vi "CheckGameBoardSnakeCheck.vi"(8 "error in (no error)":errorcluster, 11 "Board in":T3[][](array[typedef])) -> (0 "error out":errorcluster, 1 "positions":T1, 2 "Results":T2, 3 "Board out":T3[][](array[typedef]))   [LabVIEW 2020]
uses:
  TypeDef/tiles-key-trunct.ctl
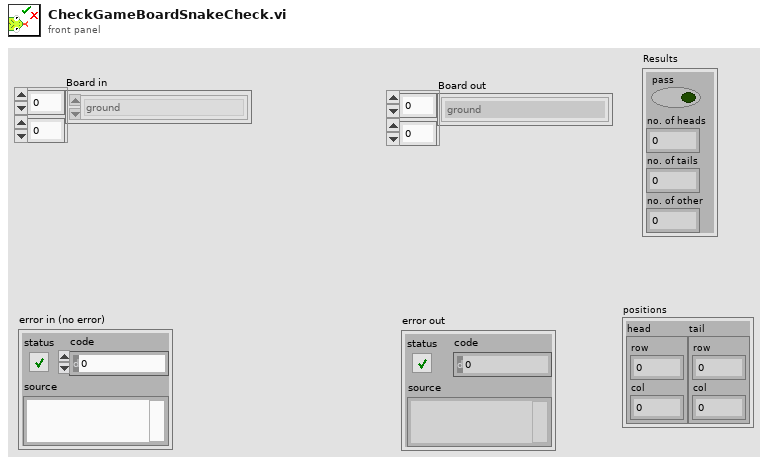
[diagram p1: front panel]
types:
  T1 = cluster{"head":cluster{"row":i32, "col":i32}, "tail":cluster{"row":i32, "col":i32}}
  T2 = cluster{"pass":bool, "no. of heads":i32, "no. of tails":i32, "no. of other":i32}
  T3 = typedef "tiles-key-trunct.ctl" = enum16{"ground", "wall", "head (right)", "head (up)", "head (left)", "head (down)", "L-turn (right-up)", "L-turn (up-left)", "L-turn (left-down)", "L-turn (down-right)", "body (right)", "body (up)", "body (left)", "body (down)", "R-turn (right-down)", "R-turn (up-right)", "R-turn (left-up)", "R-turn (down-left)", "tail (right)", "tail (up)", "tail (left)", "tail (down)"}
  T4 = typedef "direction.ctl" = enum16{"Right", "Up", "Left", "Down"}
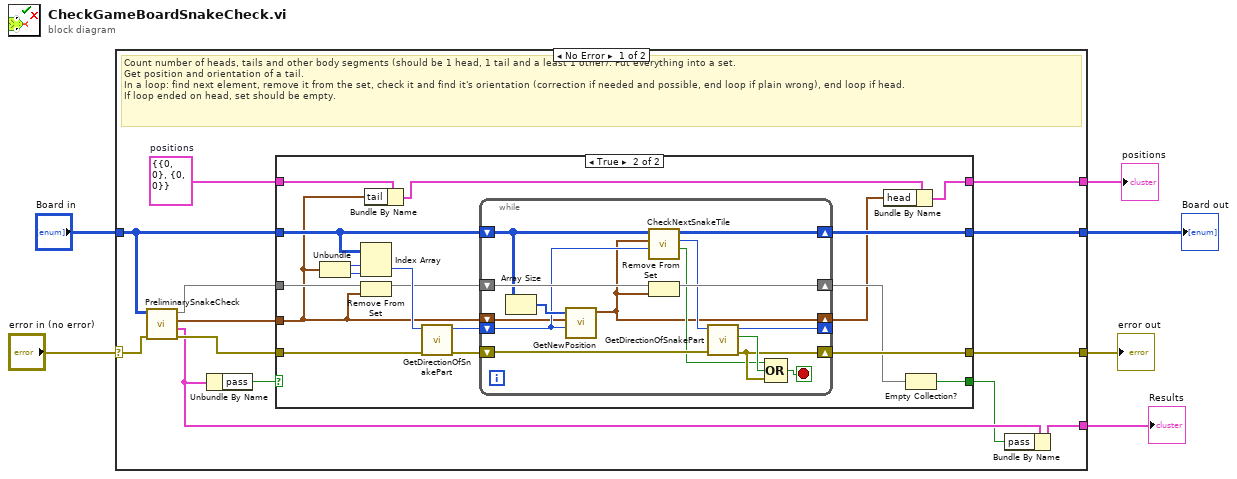
[diagram p0: block diagram]
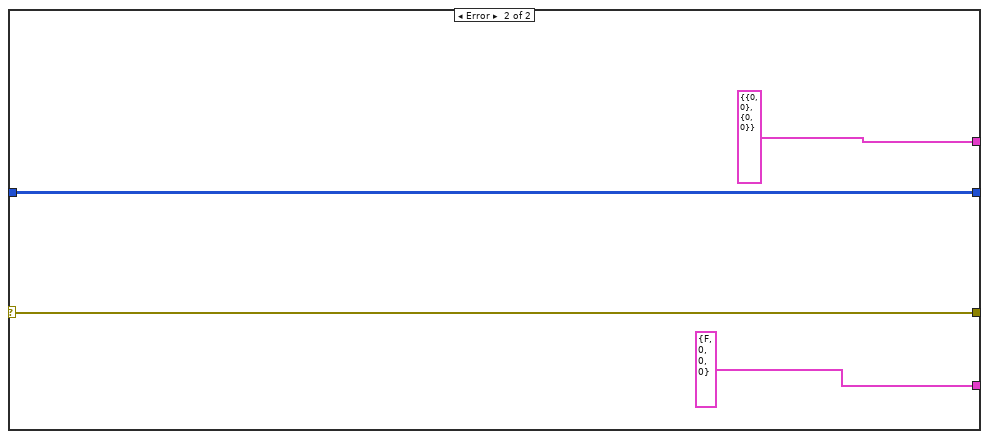
[diagram p3: hidden frame]
diagram:
  n1 = case shown="No Error" "error in (no error)" {
    selector: "error in (no error)" -> [w14 w59]
    tunnel: "Board in" -> [w18 w60]
    tunnel: [w12 w59] -> w4
    tunnel: [w19 w60] -> w3
    tunnel: [w9 T2 {"pass"=FALSE, "no. of heads"=0, "no. of tails"=0, "no. of other"=0} ("results")] -> w2
    tunnel: [w7 T1 {"head"={"row"=0, "col"=0}, "tail"={"row"=0, "col"=0}} ("positions")] -> w1
    frame No Error {
      w11 = T1 {"head"={"row"=0, "col"=0}, "tail"={"row"=0, "col"=0}}  # positions
      # "Count number of heads, tails and other body segments (should be 1 head, 1 tail and a least 1 other). Put everything into a set.\nGet position and orientation of a tail.\nIn a loop: find next element, remove it from the set, check it and find it's orientation (correction if needed and possible, end loop if plain wrong), end loop if head.\nIf loop ended on head, set should be empty."
      n2 = call "PreliminarySnakeCheck.vi"("error in (no error)"=w14, "Board in"=w18) -> ("error out"=w13:errorcluster, "results"=w10:T2, "tail position"=w15:cluster{"row":i32, "col":i32}, "bodyparts set"=w16:set{cluster{i32, i32}})  [unwired: 6 in]
      n3 = Unbundle By Name(w10) -> ("pass"=w17:bool)
      n4 = case shown="True" w17 {
        selector: w17 -> [w20 _]
        tunnel: w15 -> [_ w24]
        tunnel: w18 -> [w23 w34]
        tunnel: [w23 w41] -> w19
        tunnel: w16 -> [_ w26]
        tunnel: w13 -> [w22 w39]
        tunnel: [w22 w40] -> w12
        tunnel: w11 -> [w21 w31]
        tunnel: [w20 w28] -> w8
        tunnel: [w21 w27] -> w7
        frame False {
        }
        frame True {
          n5 = Unbundle(w24) -> ("row"=w35:i32, "col"=w36:i32)
          n6 = Index Array(array=w34, index (row)=w35, index (col)=w36) -> (element=w33:T3)
          n7 = Remove From Set(10:w24, 11:w26) -> (3:w25:set{cluster{i32, i32}})  [unwired: 1 out]
          n8 = Bundle By Name(cluster=w31, "tail"=w24) -> (w30:T1)
          n9 = call "GetDirectionOfSnakePart.vi"("error in (no error)"=w39, "tile in"=w33) -> ("error out"=w38:errorcluster, "Direction"=w37:T4)  [unwired: 7 in, 1 out]
          n10 = while {
            shift-right: [w42] -> w29
            shift-left: w24 -> [w43]
            shift-right: [w47] -> w41
            shift-left: w34 -> [w48]
            shift-right: [w55] -> w32
            shift-left: w25 -> [w56]
            shift-right: [w49] -> w40
            shift-left: w38 -> [w53]
            shift-right: [w51] -> _
            shift-left: w37 -> [w46]
            stop <- w52 stop-if-true
            n11 = Array Size(array=w48) -> (size(s)=w54:i32[])
            n12 = call "GetNewPosition.vi"("Direction"=w46, "position in"=w43, "size(s)"=w54) -> ("position out"=w42:cluster{"row":i32, "col":i32})  [unwired: 8 in]
            n13 = call "CheckNextSnakeTile.vi"("Direction (old)"=w46, "new position in"=w42, "Board in"=w48) -> ("Stop"=w44:bool, "Tile"=w45:T3, "Board out"=w47:T3[][])  [unwired: 6 in]
            n14 = Remove From Set(10:w42, 11:w56) -> (3:w55:set{cluster{i32, i32}})  [unwired: 1 out]
            n15 = call "GetDirectionOfSnakePart.vi"("error in (no error)"=w53, "tile in"=w45) -> ("error out"=w49:errorcluster, "Stop"=w50:bool, "Direction"=w51:T4)  [unwired: 7 in]
            n16 = Compound Arithmetic op=OR(w44, w50, w49) -> (w52:bool)
          }
          n17 = Bundle By Name(cluster=w30, "head"=w29) -> (w27:T1)
          n18 = Empty Collection?(1:w32) -> (0:w28:bool)
        }
      }
      n19 = Bundle By Name(cluster=w10, "pass"=w8) -> (w9:T2)
    }
    frame Error {
    }
  }
  "Board out" <- w3
  "error out" <- w4
  "Results" <- w2
  "positions" <- w1
